vi "SDCP SMF Rx Logger - Base (version 1.0).vi"() -> ()   [LabVIEW 2020]
uses:
  Typedefs/SDCP SMF Rx Logger - Notifier FGV - Notifier names.ctl
  Typedefs/SDCP SMF Rx Logger - Notifier FGV - Commands.ctl
  Typedefs/SDCP SMF logger - SMF with timestamp.ctl
  Typedefs/SDCP - Serial Port Control - Commands.ctl
panel:
  out "error out":errorcluster
  in  "error in (no error)":errorcluster
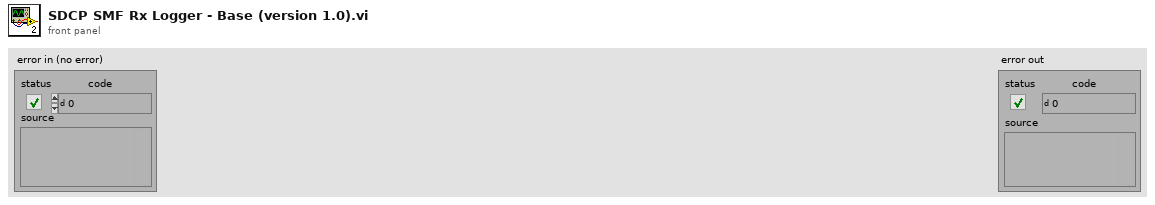
[diagram p1: front panel]
types:
  T1 = typedef "SDCP SMF Rx Logger - Notifier FGV - Commands.ctl" = enum16{"Initialize", "Read", "Write", "Deinitialize"}
  T2 = typedef "SDCP SMF Rx Logger - Notifier FGV - Notifier names.ctl" = enum16{"Logged data", "Pause logging", "Get log", "Reset log", "Stop logging"}
  T3 = typedef "SDCP SMF logger - SMF with timestamp.ctl" = cluster{"Bytes":u8[], "Checksum":bool, "Time (ms)":u32, "Tx/Rx":string}
  T4 = typedef "SDCP - Serial Port Control - Commands.ctl" = enum16{"Open", "Read", "Write", "Get instance", "Close"}
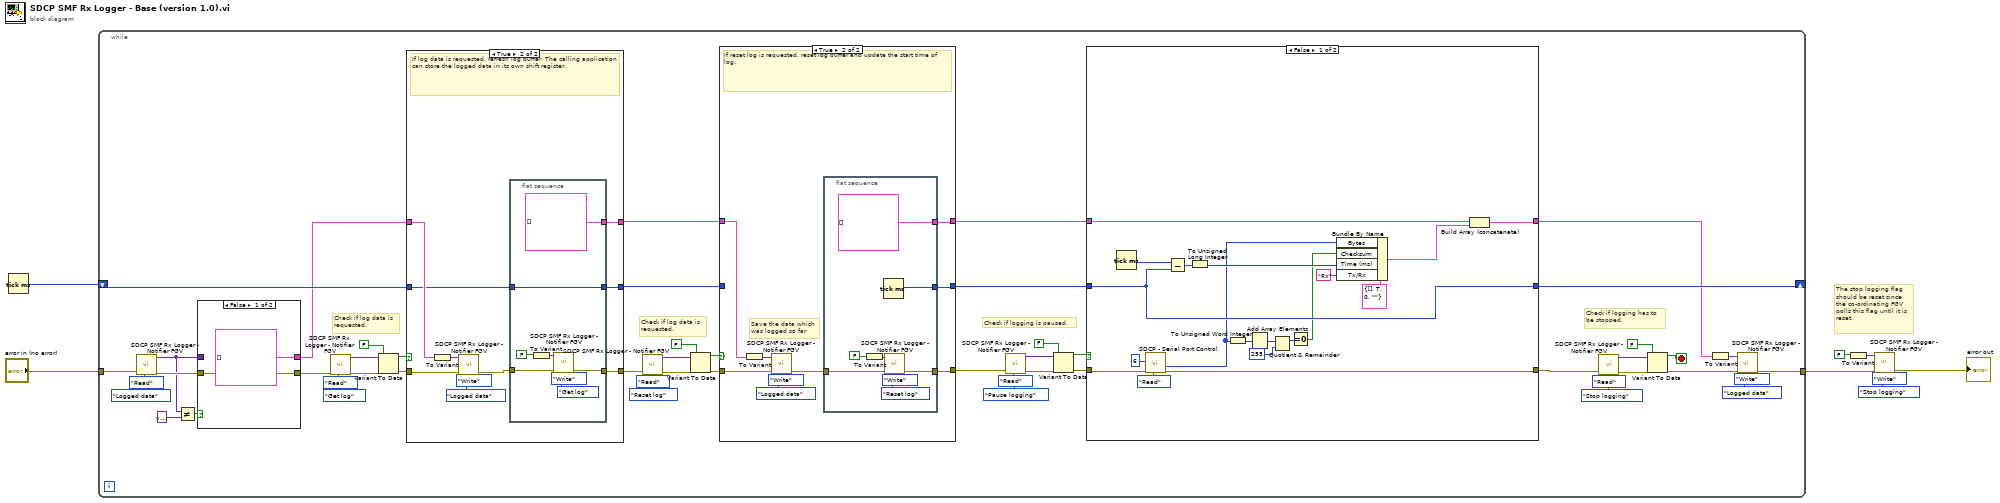
[diagram p0: block diagram]
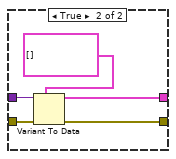
[diagram p2: hidden frame]
diagram:
  # "The stop logging flag\nshould be reset since\nthe co-ordinating FGV\npolls this flag until it is\nreset."
  n1 = Tick Count (ms)() -> (millisecond timer value=w7:u32)
  n2 = while {
    tunnel: "error in (no error)" -> [w20]
    shift-right: [w31] -> _
    shift-left: w7 -> [w59]
    tunnel: [w10] -> w1
    stop <- w24 stop-if-true
    # "Check if logging has to\nbe stopped."
    # "Check if logging is paused."
    # "Check if log data is\nrequested."
    # "Check if log data is\nrequested."
    n3 = call "SDCP SMF Rx Logger - Notifier FGV.vi"("error in (no error)"=w20, "Command"=SDCP_SMF_Rx_Logger_-_Notifier_FGV_-_Commands."Read", "Notifier name"=SDCP_SMF_Rx_Logger_-_Notifier_FGV_-_Notifier_names."Logged data") -> ("error out"=w23:errorcluster, "Notifier value out"=w18:variant)  [unwired: 3 in]
    n4 = Not Equal?(x=w18, y=variant) -> (x != y?=w19:bool)
    n5 = case shown="False" w19 {
      tunnel: w23 -> [w61 w66]
      tunnel: w18 -> [_ w65]
      tunnel: [w61 w63] -> w16
      tunnel: [T3[] [] w62] -> w15
      frame False {
      }
      frame True {
        n6 = Variant To Data(error in=w66, type=T3[] [], Variant=w65) -> (data=w62:T3[], error out=w63:errorcluster)
      }
    }
    n7 = call "SDCP SMF Rx Logger - Notifier FGV.vi"("error in (no error)"=w16, "Command"=SDCP_SMF_Rx_Logger_-_Notifier_FGV_-_Commands."Read", "Notifier name"=SDCP_SMF_Rx_Logger_-_Notifier_FGV_-_Notifier_names."Get log") -> ("error out"=w58:errorcluster, "Notifier value out"=w57:variant)  [unwired: 3 in]
    n8 = Variant To Data(error in=w58, type=FALSE, Variant=w57) -> (data=w54:bool, error out=w55:errorcluster)
    n9 = case shown="True" w54 {
      tunnel: w55 -> [w111 w121]
      tunnel: w15 -> [w109 w119]
      tunnel: [w111 w115] -> w44
      tunnel: w59 -> [w110 w113]
      tunnel: [w110 w112] -> w43
      tunnel: [w109 w114] -> w42
      frame False {
      }
      frame True {
        # "If log data is requested, refresh log buffer. The calling application can store the logged data in its own shift register."
        n10 = To Variant(anything=w119) -> (Variant=w120:variant)
        n11 = call "SDCP SMF Rx Logger - Notifier FGV.vi"("error in (no error)"=w121, "Command"=SDCP_SMF_Rx_Logger_-_Notifier_FGV_-_Commands."Write", "Notifier name"=SDCP_SMF_Rx_Logger_-_Notifier_FGV_-_Notifier_names."Logged data", "Notifier value in"=w120) -> ("error out"=w116:errorcluster)  [unwired: 2 in, 1 out]
        n12 = flat-sequence {
          tunnel: w116 -> [w126]
          tunnel: [w124] -> w115
          tunnel: [T3[] []] -> w114
          tunnel: w113 -> [w122]
          tunnel: [w122] -> w112
          frame #0 {
            n13 = To Variant(anything=FALSE) -> (Variant=w129:variant)
            n14 = call "SDCP SMF Rx Logger - Notifier FGV.vi"("error in (no error)"=w126, "Command"=SDCP_SMF_Rx_Logger_-_Notifier_FGV_-_Commands."Write", "Notifier name"=SDCP_SMF_Rx_Logger_-_Notifier_FGV_-_Notifier_names."Get log", "Notifier value in"=w129) -> ("error out"=w124:errorcluster)  [unwired: 2 in, 1 out]
          }
        }
      }
    }
    n15 = call "SDCP SMF Rx Logger - Notifier FGV.vi"("error in (no error)"=w44, "Command"=SDCP_SMF_Rx_Logger_-_Notifier_FGV_-_Commands."Read", "Notifier name"=SDCP_SMF_Rx_Logger_-_Notifier_FGV_-_Notifier_names."Reset log") -> ("error out"=w51:errorcluster, "Notifier value out"=w50:variant)  [unwired: 3 in]
    n16 = Variant To Data(error in=w51, type=FALSE, Variant=w50) -> (data=w47:bool, error out=w48:errorcluster)
    n17 = case shown="True" w47 {
      tunnel: w48 -> [w91 w100]
      tunnel: w42 -> [w89 w98]
      tunnel: [w91 w94] -> w36
      tunnel: w43 -> [w90 _]
      tunnel: [w90 w93] -> w32
      tunnel: [w89 w92] -> w33
      frame False {
      }
      frame True {
        # "Save the data which\nwas logged so far"
        # "If reset log is requested, reset log buffer and update the start time of log."
        n18 = To Variant(anything=w98) -> (Variant=w99:variant)
        n19 = call "SDCP SMF Rx Logger - Notifier FGV.vi"("error in (no error)"=w100, "Command"=SDCP_SMF_Rx_Logger_-_Notifier_FGV_-_Commands."Write", "Notifier name"=SDCP_SMF_Rx_Logger_-_Notifier_FGV_-_Notifier_names."Logged data", "Notifier value in"=w99) -> ("error out"=w95:errorcluster)  [unwired: 2 in, 1 out]
        n20 = flat-sequence {
          tunnel: w95 -> [w105]
          tunnel: [w103] -> w94
          tunnel: [w102] -> w93
          tunnel: [T3[] []] -> w92
          frame #0 {
            n21 = To Variant(anything=FALSE) -> (Variant=w108:variant)
            n22 = Tick Count (ms)() -> (millisecond timer value=w102:u32)
            n23 = call "SDCP SMF Rx Logger - Notifier FGV.vi"("error in (no error)"=w105, "Command"=SDCP_SMF_Rx_Logger_-_Notifier_FGV_-_Commands."Write", "Notifier name"=SDCP_SMF_Rx_Logger_-_Notifier_FGV_-_Notifier_names."Reset log", "Notifier value in"=w108) -> ("error out"=w103:errorcluster)  [unwired: 2 in, 1 out]
          }
        }
      }
    }
    n24 = call "SDCP SMF Rx Logger - Notifier FGV.vi"("error in (no error)"=w36, "Command"=SDCP_SMF_Rx_Logger_-_Notifier_FGV_-_Commands."Read", "Notifier name"=SDCP_SMF_Rx_Logger_-_Notifier_FGV_-_Notifier_names."Pause logging") -> ("error out"=w41:errorcluster, "Notifier value out"=w40:variant)  [unwired: 3 in]
    n25 = Variant To Data(error in=w41, type=FALSE, Variant=w40) -> (data=w34:bool, error out=w35:errorcluster)
    n26 = case shown="False" w34 {
      tunnel: w35 -> [w85 w86]
      tunnel: w33 -> [w77 w88]
      tunnel: [w75 w88] -> w9
      tunnel: w32 -> [w74 w87]
      tunnel: [w74 w87] -> w31
      tunnel: [w73 w86] -> w25
      frame False {
        n27 = Tick Count (ms)() -> (millisecond timer value=w81:u32)
        n28 = call "SDCP - Serial Port Control.vi"("Command"=SDCP_-_Serial_Port_Control_-_Commands."Read", "error in (no error)"=w85, "Read byte count"=u32 6) -> ("error out"=w73:errorcluster, "Received bytes"=w72:u8[])  [unwired: 7 in]
        n29 = Subtract(x=w81, y=w74) -> (x-y=w80:u32)
        n30 = To Unsigned Long Integer(number=w80) -> (unsigned 32bit integer=w79:u32)
        n31 = To Unsigned Word Integer(number=w72) -> (unsigned 16bit integer=w71:u16[])
        n32 = Add Array Elements(numeric array=w71) -> (sum=w70:u16)
        n33 = Quotient & Remainder(x=w70, y=u16 255) -> (x-y*floor(x/y)=w68:u16)  [unwired: 1 out]
        n34 = Equal To 0?(x=w68) -> (x = 0?=w67:bool)
        n35 = Bundle By Name(cluster=T3 {"Bytes"=[], "Checksum"=TRUE, "Time (ms)"=0, "Tx/Rx"=""} ("SMF with timestamp"), "Bytes"=w72, "Checksum"=w67, "Time (ms)"=w79, "Tx/Rx"="Rx") -> (w76:T3)
        n36 = Build Array (concatenate)(w77, w76) -> (w75:T3[])
      }
      frame True {
        # "Logging is paused. Do nothing."
      }
    }
    n37 = call "SDCP SMF Rx Logger - Notifier FGV.vi"("error in (no error)"=w25, "Command"=SDCP_SMF_Rx_Logger_-_Notifier_FGV_-_Commands."Read", "Notifier name"=SDCP_SMF_Rx_Logger_-_Notifier_FGV_-_Notifier_names."Stop logging") -> ("error out"=w30:errorcluster, "Notifier value out"=w29:variant)  [unwired: 3 in]
    n38 = Variant To Data(error in=w30, type=FALSE, Variant=w29) -> (data=w24:bool, error out=w11:errorcluster)
    n39 = To Variant(anything=w9) -> (Variant=w14:variant)
    n40 = call "SDCP SMF Rx Logger - Notifier FGV.vi"("error in (no error)"=w11, "Command"=SDCP_SMF_Rx_Logger_-_Notifier_FGV_-_Commands."Write", "Notifier name"=SDCP_SMF_Rx_Logger_-_Notifier_FGV_-_Notifier_names."Logged data", "Notifier value in"=w14) -> ("error out"=w10:errorcluster)  [unwired: 2 in, 1 out]
  }
  n41 = To Variant(anything=FALSE) -> (Variant=w6:variant)
  n42 = call "SDCP SMF Rx Logger - Notifier FGV.vi"("error in (no error)"=w1, "Command"=SDCP_SMF_Rx_Logger_-_Notifier_FGV_-_Commands."Write", "Notifier name"=SDCP_SMF_Rx_Logger_-_Notifier_FGV_-_Notifier_names."Stop logging", "Notifier value in"=w6) -> ("error out"=→"error out":errorcluster)  [unwired: 2 in, 1 out]
